vi "flushQueueTcpClient.vi"(8 "error in (no error)":errorcluster, 11 "TcpServerBase in":refnum<class "TcpServerBase.lvclass">) -> (0 "error out":errorcluster, 3 "TcpServerBase out":refnum<class "TcpServerBase.lvclass">)   [LabVIEW 2018, in "TcpServerBase.lvclass"]
doc: "Flush queueTcpClient when TCP client is unconnected and there are still elements in the queue."
uses:
  TcpServerBase.lvclass
  TcpServerBase.lvclass/TcpServerBase.ctl
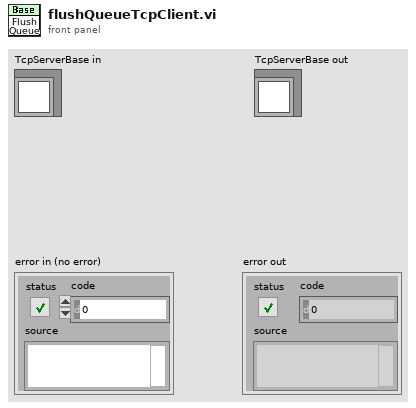
[diagram p1: front panel]
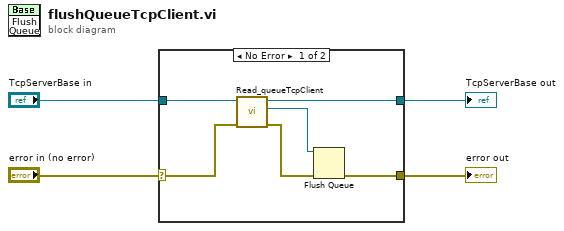
[diagram p0: block diagram]
diagram:
  n1 = case shown="No Error" "error in (no error)" {
    selector: "error in (no error)" -> [w8 w11]
    tunnel: "TcpServerBase in" -> [w10 w12]
    tunnel: [w9 w12] -> w2
    tunnel: [w5 w11] -> w1
    frame No Error {
      n2 = call "Read_queueTcpClient.vi"("error in (no error)"=w8, "TcpServerBase in"=w10) -> ("error out"=w6:errorcluster, "queueTcpClient"=w7:refnum<queue>, "TcpServerBase out"=w9:refnum<class "TcpServerBase.lvclass">)  [unwired: 7 in]
      n3 = Flush Queue(queue=w7, error in (no error)=w6) -> (error out=w5:errorcluster)  [unwired: 2 out]
    }
    frame Error {
    }
  }
  "error out" <- w1
  "TcpServerBase out" <- w2
